vi "load-from-atlas.vi"(9 "slice":u32, 10 "image width":i32, 11 "Data TIFF File":path) -> (3 "buffer":sgl[](array[numeric]))   [LabVIEW 2013]
uses:
  imagereconstruction/x64/Debug/labviewdll.dll
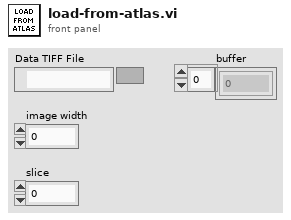
[diagram p1: front panel]
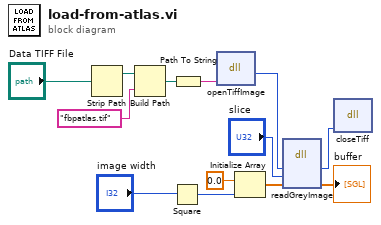
[diagram p0: block diagram]
diagram:
  n1 = Strip Path(path="Data TIFF File") -> (stripped path=w2:path)  [unwired: 1 out]
  n2 = Build Path(base path=w2, name or relative path="fbpatlas.tif") -> (appended path=w1:path)
  n3 = Square(x="image width") -> (x^2=w9:i32)
  n4 = Path To String(path=w1) -> (string=w5:string)
  n5 = dll-call lib="D:/work/uni/FYP/reconrepo/imagereconstruction/x64/Debug/labviewdll.dll" fn="openTiffImage"("pathname"=w5) -> ("tiff"=w6:i64)  [unwired: 4 in, 2 out]
  n6 = Initialize Array(sgl 0.0 ("element"), w9) -> (w11:sgl[])
  n7 = dll-call lib="D:/work/uni/FYP/reconrepo/imagereconstruction/x64/Debug/labviewdll.dll" fn="readGreyImage"("tiff"=w6, "directory"="slice", "buffer"=w11) -> ("tiff"=w13:i64, "buffer"=→"buffer":sgl[])  [unwired: 5 in, 2 out]
  n8 = dll-call lib="D:/work/uni/FYP/reconrepo/imagereconstruction/x64/Debug/labviewdll.dll" fn="closeTiff"("tiff"=w13) -> ()  [unwired: 5 in, 2 out]
